vi "filter to finite value.vi"(1 "filters":T1={"infinity"=TRUE, "- infinity"=TRUE, "NaN"=TRUE, "zero"=FALSE}, 2 "replacement value":dbl, 3 "value":dbl) -> (0 "filtered value":dbl)   [LabVIEW 2009]
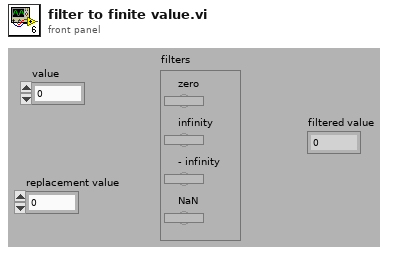
[diagram p1: front panel]
types:
  T1 = cluster{"infinity":bool, "- infinity":bool, "NaN":bool, "zero":bool}
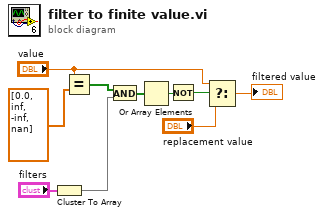
[diagram p0: block diagram]
diagram:
  n1 = Cluster To Array(cluster="filters") -> (array=w8:bool[])
  n2 = Equal?(x="value", y=dbl[] [0.0, inf, -inf, nan]) -> (x = y?=w7:bool[])
  n3 = And(x=w7, y=w8) -> (x .and. y?=w6:bool[])
  n4 = Or Array Elements(Boolean array=w6) -> (logical OR=w5:bool)
  n5 = Not(x=w5) -> (.not. x?=w4:bool)
  n6 = Select(t="value", s=w4, f="replacement value") -> (s? t:f=→"filtered value":dbl)
